vi "Find autonmous program from name.vi"(10 "Program Name":string, 11 "All Autonmous Programs":T3) -> (2 "did it find it?":bool, 3 "Autonmous Program":T1)   [LabVIEW 2013]
uses:
  All Autonmous Programs typedef.ctl
  Autonmous Program typedef.ctl
  Autonmous Scripting array typedef.ctl
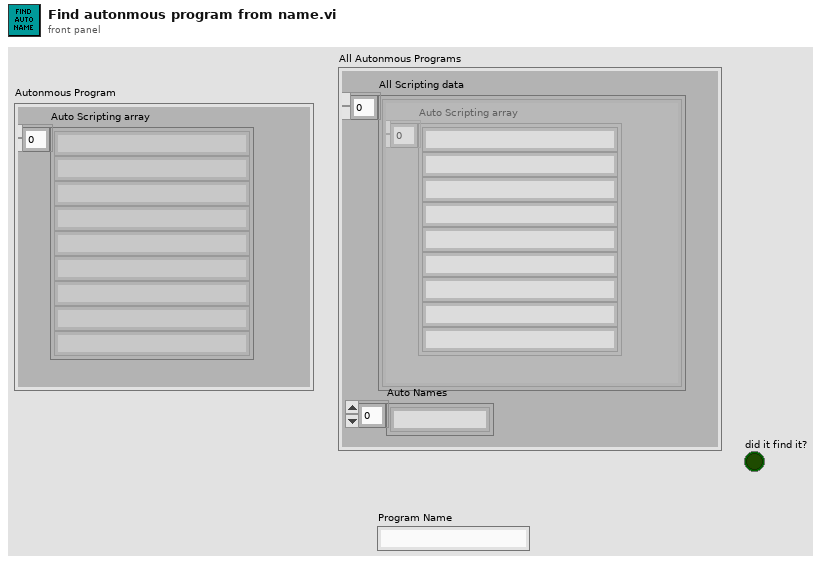
[diagram p1: front panel]
types:
  T1 = typedef "Autonmous Program typedef.ctl" = cluster{"Auto Scripting array":T2}
  T2 = typedef "Autonmous Scripting array typedef.ctl" = string[]
  T3 = typedef "All Autonmous Programs typedef.ctl" = cluster{"All Scripting data":T1[], "Auto Names":string[]}
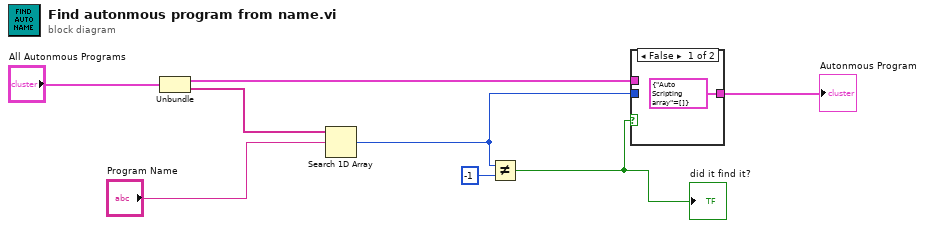
[diagram p0: block diagram]
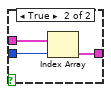
[diagram p2: hidden frame]
diagram:
  n1 = Unbundle("All Autonmous Programs") -> ("All Scripting data"=w4:T1[], "Auto Names"=w5:string[])
  n2 = Search 1D Array(1D array=w5, element="Program Name") -> (index of element=w3:i32)  [unwired: 1 in]
  n3 = Not Equal?(x=w3, y=-1) -> (x != y?=w6:bool)
  "did it find it?" <- w6
  n4 = case shown="False" w6 {
    tunnel: w3 -> [_ w11]
    tunnel: w4 -> [_ w12]
    tunnel: [T1 {"Auto Scripting array"=[]} ("Autonmous Program") w10] -> w1
    frame False {
    }
    frame True {
      n5 = Index Array(array=w12, index=w11) -> (element=w10:T1)
    }
  }
  "Autonmous Program" <- w1
